vi "Inject Teller Metadata.vi"(4 "Priority":bool, 8 "Error in":errorcluster, 9 "Reply":bool, 10 "Msg":refnum<class "Msg.lvclass">, 11 "TEMPLATE Actor in":refnum<class "TEMPLATE Actor.lvclass">) -> (2 "Teller Metadata":refnum<class "Teller Metadata.lvclass">)   [LabVIEW 2025, in "_Template.lvlib" / "Templates.lvlib" / "TEMPLATE jettl Actor.lvlib" / "TEMPLATE Actor.lvlib" / "TEMPLATE Actor.lvclass"]
uses:
  TEMPLATE Actor.lvclass
  jettl/jettl/Teller Metadata/Teller Metadata.lvclass
  jettl/jettl/Msg/Msg.lvclass
  jettl/jettl/jettl.lvlib
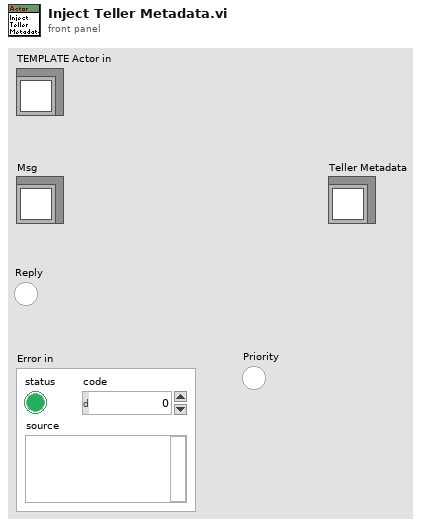
[diagram p1: front panel]
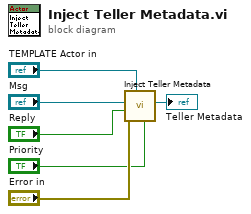
[diagram p0: block diagram]
diagram:
  n1 = call "Inject Teller Metadata.vi"("Priority"="Priority", "Actor in"="TEMPLATE Actor in", "Error in"="Error in", "Reply"="Reply", "Msg"="Msg") -> ("Teller Metadata"=→"Teller Metadata":refnum<class "Teller Metadata.lvclass">)  [unwired: 6 in]
